vi "Read.vi"(8 "error in (no error)":errorcluster, 11 "Maxon Encoder in":refnum<class "Maxon Encoder.lvclass">) -> (0 "error out":errorcluster, 1 "Velocity (rad/Sec)":dbl, 2 "Angular Position (rad)":dbl, 3 "Maxon Encoder out":refnum<class "Maxon Encoder.lvclass">)   [LabVIEW 2019, in "Maxon Encoder.lvclass"]
doc: "Reads the angular position in degrees."
uses:
  Maxon Encoder.lvclass
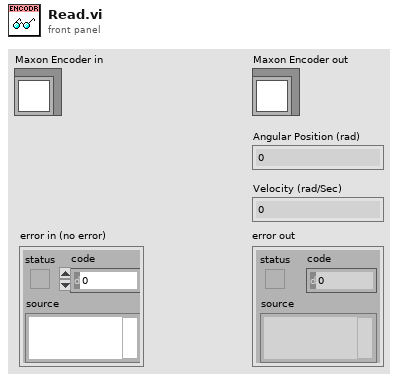
[diagram p1: front panel]
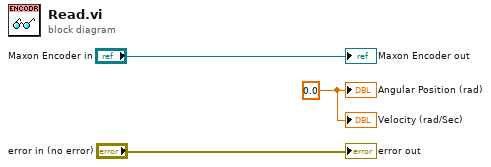
[diagram p0: block diagram]
diagram:
  w1 = 0.0 ("Angular Position (rad)")
  "error out" <- "error in (no error)"
  "Angular Position (rad)" <- w1
  "Maxon Encoder out" <- "Maxon Encoder in"
  "Velocity (rad/Sec)" <- w1
